vi "SoundMaxDetect_subvi.vi"(10 "Threshold":dbl, 11 "Buffer In":dbl[](array[numeric])) -> (1 "Just Changed":bool, 2 "Max Found":bool, 3 "Peak Index":i32)   [LabVIEW 2019]
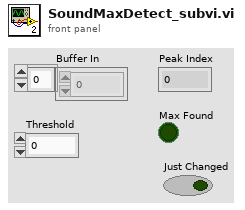
[diagram p1: front panel]
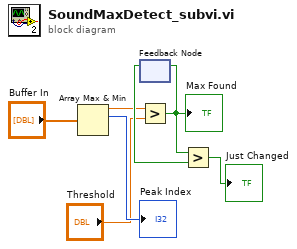
[diagram p0: block diagram]
diagram:
  n1 = Array Max & Min(array="Buffer In") -> (max value=w3:dbl, max index (indices)=→"Peak Index":i32)  [unwired: 2 out]
  n2 = feedback #1() -> (w5:bool)  [unwired: 1 in]
  n3 = Greater?(x=w3, y="Threshold") -> (0:w4:bool)
  "Max Found" <- w4
  n4 = feedback-in #1(w4) -> ()
  n5 = Greater?(x=w4, y=w5) -> (0:→"Just Changed":bool)
